vi "Actor Core.vi"(8 "error in":errorcluster, 11 "UDP_Service in":refnum<class "UDP_Service.lvclass">) -> (0 "error out":errorcluster, 3 "Actor out":refnum<class "Actor.lvclass">)   [LabVIEW 2016, in "CoreAssertAPI.lvlib" / "UDP_Service.lvclass"]
doc: "(<B>Filename</B>: Actor Framework.lvlib:Actor.lvclass:Actor Core.vi)\n\nReceives messages to the actor, reacts to them, and initiates any error handling that may shut the actor down.\n\nDescendant classes may override this VI to append parallel tasks for the actor to complete while it handles messages. Overrides use the Call Parent Method node."
uses:
  UDP_Service.lvclass
  <vilib>/ActorFramework/Actor/Actor.lvclass
  UDP_Service.lvclass/UDP_Service.ctl
  Assert Packet.ctl
  Message Data.ctl
  VI References.ctl
  CoreAssertAPI.lvlib
panel:
  out "IP Address":string
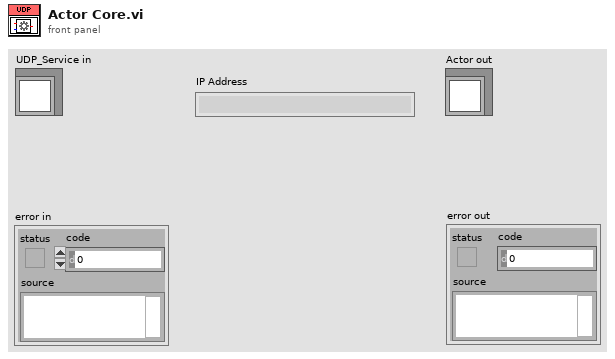
[diagram p1: front panel]
types:
  T1 = typedef "CoreAssertAPI.lvlib/Assert Packet.ctl" = cluster{"Assert Message":T2}
  T2 = typedef "CoreAssertAPI.lvlib/Message Data.ctl" = cluster{"Data Value":variant, "Last Update":timestamp, "Comment":string, "Evaluation String":string, "Status":string, "Assert Name":string, "Failure Action":string, "Assert VI Name":string, "Calling VI Name":string, "Assert VI UID":i32, "Top Level VI Name":string, "VI References":T3, "Assert Build Timestamp":timestamp, "Assert Builder User Name":string, "Data Type":string}
  T3 = typedef "CoreAssertAPI.lvlib/VI References.ctl" = cluster{"Calling VI Ref":refnum<vi>, "Assert VI Ref":refnum<vi>}
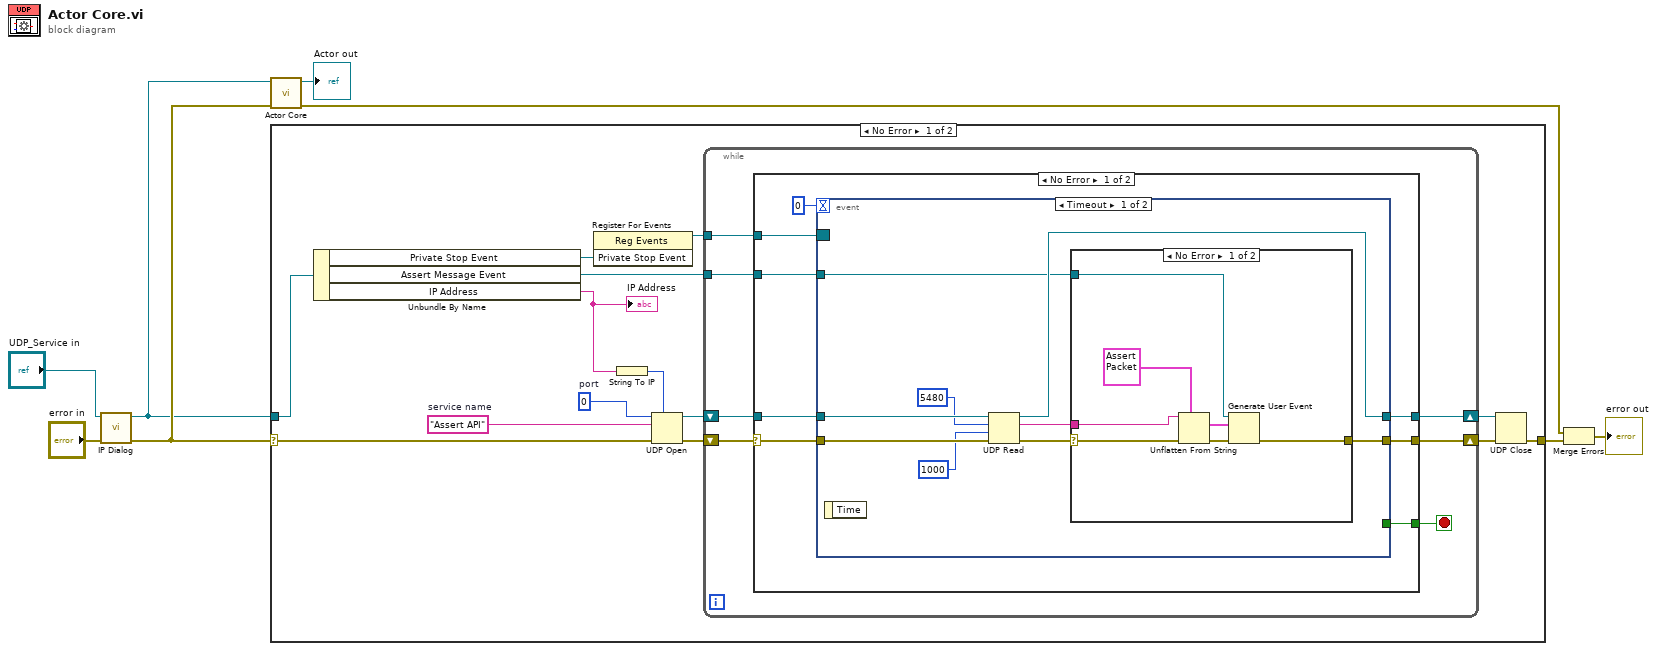
[diagram p0: block diagram]
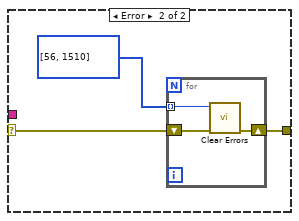
[diagram p2: hidden frame]
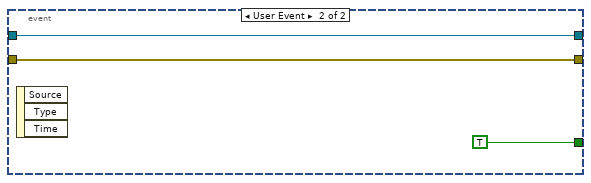
[diagram p3: hidden frame]
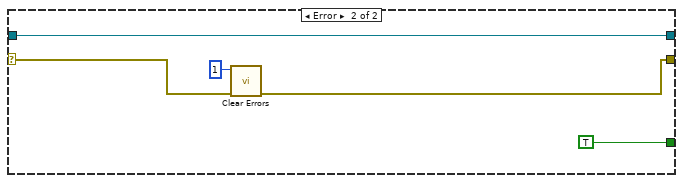
[diagram p4: hidden frame]
diagram:
  n1 = call "IP Dialog.vi"("error in (no error)"="error in", "UDP_Service in"="UDP_Service in") -> ("error out"=w4:errorcluster, "UDP_Service out"=w3:refnum<class "UDP_Service.lvclass">)  [unwired: 8 in]
  n2 = call-parent "Actor Core.vi"("error in"=w4, "Actor in"=w3) -> ("error out"=w8:errorcluster, "Actor out"=→"Actor out":refnum<class "Actor.lvclass">)  [unwired: 8 in]
  n3 = case shown="No Error" w4 {
    selector: w4 -> [w13 w68]
    tunnel: w3 -> [w15 _]
    tunnel: [w12 w68] -> w1
    frame No Error {
      w10 = "Assert API"  # service name
      w18 = u16 0  # port
      n4 = Unbundle By Name(w15) -> ("Private Stop Event"=w14:refnum<user-event>, "Assert Message Event"=w21:refnum<user-event>, "IP Address"=w11:string)
      "IP Address" <- w11
      n5 = register-events(w14) -> (reference out=w22:refnum<event-registration>)  [unwired: 2 in, 1 out]
      n6 = String To IP(1:w11) -> (0:w9:u32)
      n7 = UDP Open(7:w9, 8:w13, 10:w10, 11:w18) -> (port=w19:refnum<k16>, 0:w20:errorcluster)  [unwired: 1 in, 1 out]
      n8 = while {
        shift-right: [w28] -> w17
        shift-left: w19 -> [w27]
        shift-right: [w29] -> w16
        shift-left: w20 -> [w26]
        tunnel: w21 -> [w25]
        tunnel: w22 -> [w24]
        stop <- w23 stop-if-true
        n9 = case shown="No Error" w26 {
          selector: w26 -> [w34 w65]
          tunnel: [w37 w63] -> w29
          tunnel: [w36 w67] -> w28
          tunnel: w27 -> [w35 w67]
          tunnel: w25 -> [w33 _]
          tunnel: w24 -> [w32 _]
          tunnel: [w31 TRUE] -> w23
          frame No Error {
            n10 = event shown="[0] Timeout" {
              selector: w32 -> [_ _]
              dyn-events: _ -> [_ _]
              timeout: 0 -> [_ _]
              tunnel: [w42 w61] -> w37
              tunnel: [w46 w60] -> w36
              tunnel: w35 -> [w45 w60]
              tunnel: w34 -> [w44 w61]
              tunnel: w33 -> [w43 _]
              tunnel: [_ TRUE] -> w31
              event Timeout {
                n11 = event-data() -> ()  [unwired: 1 in, 1 out]
                n12 = UDP Read(connection ID=w45, max size (548)=5480, timeout ms (25000)=1000, 8:w44) -> (data out=w39:string, error out=w38:errorcluster, 3:w46:refnum<k16>)  [unwired: 2 out]
                n13 = case shown="No Error" w38 {
                  selector: w38 -> [w51 w55]
                  tunnel: w43 -> [w53 _]
                  tunnel: [w52 w54] -> w42
                  tunnel: w39 -> [w47 _]
                  frame No Error {
                    n14 = Unflatten From String(type=T1 {"Assert Message"={"Data Value"=variant, "Last Update"=timestamp(0 s since 1904-01-01), "Comment"="", "Evaluation String"="", "Status"="", "Assert Name"="", "Failure Action"="", "Assert VI Name"="", "Calling VI Name"="", "Assert VI UID"=0, "Top Level VI Name"="", "VI References"={"Calling VI Ref"=refnum, "Assert VI Ref"=refnum}, "Assert Build Timestamp"=timestamp(0 s since 1904-01-01), "Assert Builder User Name"="", "Data Type"=""}} ("event data"), binary string=w47, error in (no error)=w51) -> (value=w50:T1, error out=w49:errorcluster)  [unwired: 2 in, 1 out]
                    n15 = Generate User Event(user event=w53, event data cluster=w50, error in=w49) -> (error out=w52:errorcluster)  [unwired: 1 in, 1 out]
                  }
                  frame Error {
                    n16 = for {
                      tunnel: i32[] [56, 1510] ("specific error code to clear (0: all)") -> [w59] mode=indexing
                      shift-right: [w57] -> w54
                      shift-left: w55 -> [w58]
                      n17 = call <vilib>:"Clear Errors.vi"("error in (no error)"=w58, "specific error code to clear (0: all)"=w59) -> ("error out"=w57:errorcluster)  [unwired: 4 in, 1 out]
                    }
                  }
                }
              }
              event User Event {
                n18 = event-data() -> ()  [unwired: 1 in, 3 out]
              }
            }
          }
          frame Error {
            n19 = call <vilib>:"Clear Errors.vi"("error in (no error)"=w65, "specific error code to clear (0: all)"=1) -> ("error out"=w63:errorcluster)  [unwired: 4 in, 1 out]
          }
        }
      }
      n20 = UDP Close(connection ID=w17, 8:w16) -> (error out=w12:errorcluster)  [unwired: 1 out]
    }
    frame Error {
    }
  }
  n21 = Merge Errors(w8, w1) -> (→"error out":errorcluster)
